vi "Practica_1y2_Punto_3_3.vi"() -> ()   [LabVIEW 2020]
panel:
  out "XY Graph":cluster{dbl[], dbl[]}(graph)
  in  "B":dbl
  in  "A":dbl
  out "Array":dbl[](array[numeric])
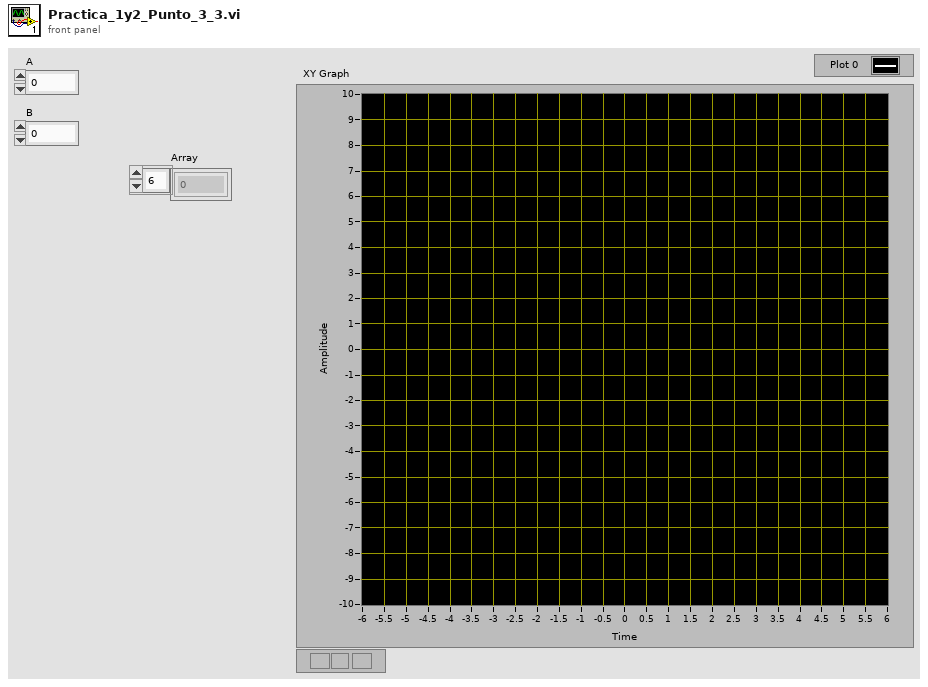
[diagram p1: front panel]
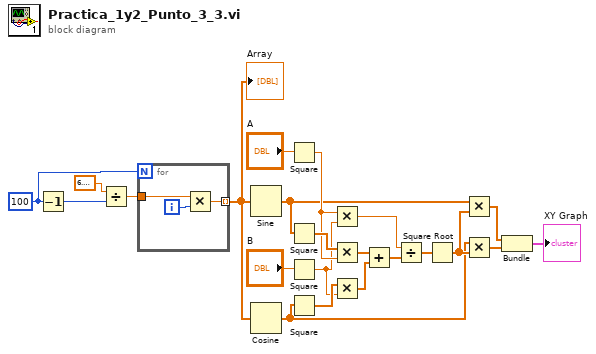
[diagram p0: block diagram]
diagram:
  w21 = 100
  n1 = Decrement(x=w21) -> (x-1=w1:i32)
  n2 = Divide(x=6.283185307179586, y=w1) -> (x/y=w2:dbl)
  n3 = for {
    N: w21 -> [_]
    tunnel: w2 -> [w25]
    tunnel: [w23] -> w20 mode=indexing
    i -> [w24]
    n4 = Multiply(x=w25, y=w24) -> (x*y=w23:dbl)
  }
  "Array" <- w20
  n5 = Sine(x=w20) -> (sin(x)=w7:dbl[])
  n6 = Cosine(x=w20) -> (cos(x)=w6:dbl[])
  n7 = Square(x="A") -> (x^2=w15:dbl)
  n8 = Square(x=w7) -> (x^2=w16:dbl[])
  n9 = Square(x="B") -> (x^2=w14:dbl)
  n10 = Square(x=w6) -> (x^2=w17:dbl[])
  n11 = Multiply(x=w15, y=w14) -> (x*y=w11:dbl)
  n12 = Multiply(x=w16, y=w15) -> (x*y=w13:dbl[])
  n13 = Multiply(x=w17, y=w14) -> (x*y=w12:dbl[])
  n14 = Add(x=w13, y=w12) -> (x+y=w10:dbl[])
  n15 = Divide(x=w11, y=w10) -> (x/y=w9:dbl[])
  n16 = Square Root(x=w9) -> (sqrt(x)=w8:dbl[])
  n17 = Multiply(x=w7, y=w8) -> (x*y=w5:dbl[])
  n18 = Multiply(x=w6, y=w8) -> (x*y=w4:dbl[])
  n19 = Bundle(w5, w4) -> (→"XY Graph":cluster{dbl[], dbl[]})  [unwired: 1 in]
